vi "下载查询数据库.vi"(8 "时间标识":timestamp=timestamp(3675413438.482 s since 1904-01-01), 9 "Row name":string="13131", 10 "pathcheck选项":T1, 11 "数据库操作选项":T2) -> (0 "OK":bool, 1 "Columns":string[](array[string]), 2 "Results":string[][](array[string]), 3 "Tables":string[](array[string]))   [LabVIEW 2017]
uses:
  Sqlite/CBB/ReadAllData.vi
  <vilib>/Utility/file.llb/Write Delimited Spreadsheet (string).vi
  Sqlite/CBB/DeleteRow.vi
  Sqlite/SQLite.lvlib
  Sqlite/CBB/DropTable.vi
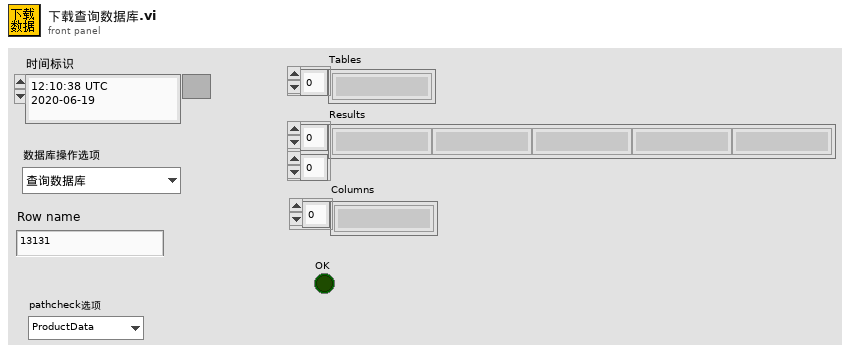
[diagram p1: front panel]
types:
  T1 = typedef "pathcheck选项.ctl" = enum16{"ProductData", "CTData", "ERData", "IOTDATA"}
  T2 = typedef "数据库操作选项.ctl" = enum16{"查询数据库", "下载数据", "删除table", "删除数据库对应行"}
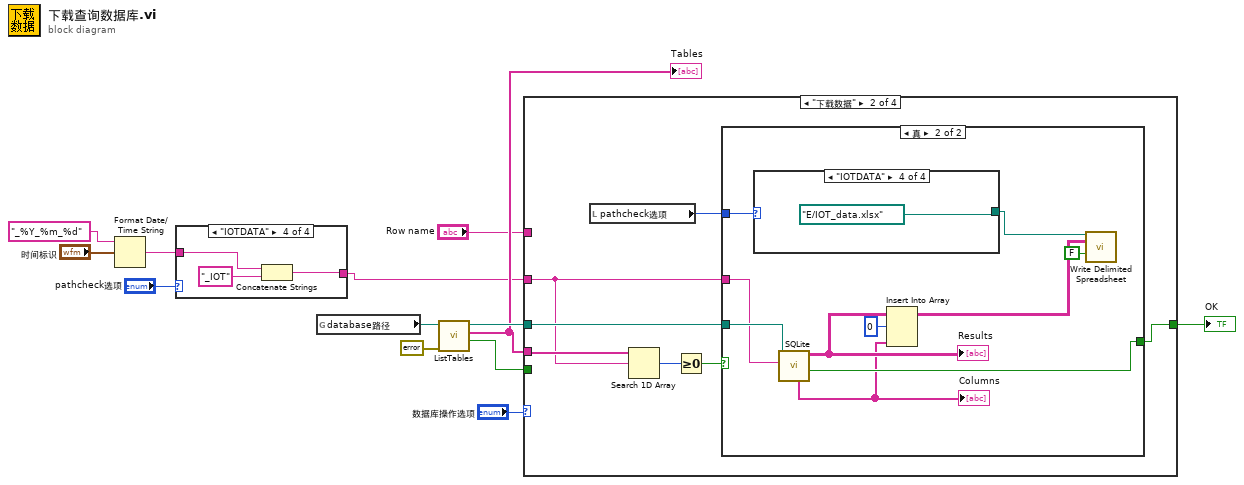
[diagram p0: block diagram]
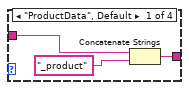
[diagram p2: hidden frame]
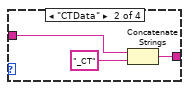
[diagram p3: hidden frame]
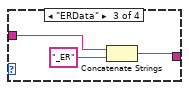
[diagram p4: hidden frame]
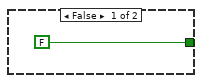
[diagram p6: hidden frame]
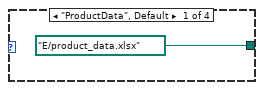
[diagram p7: hidden frame]
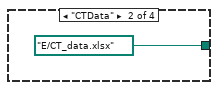
[diagram p8: hidden frame]
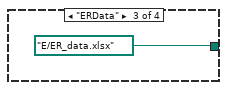
[diagram p9: hidden frame]
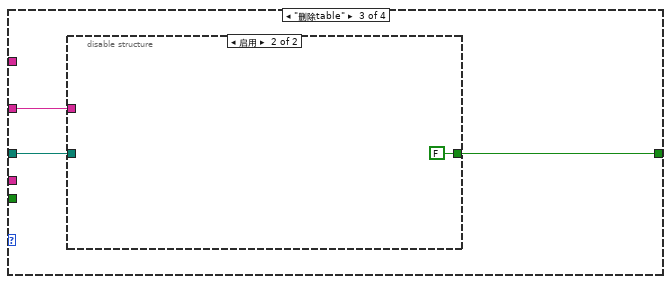
[diagram p10: hidden frame]
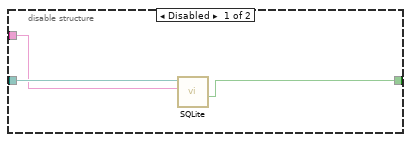
[diagram p11: hidden frame]
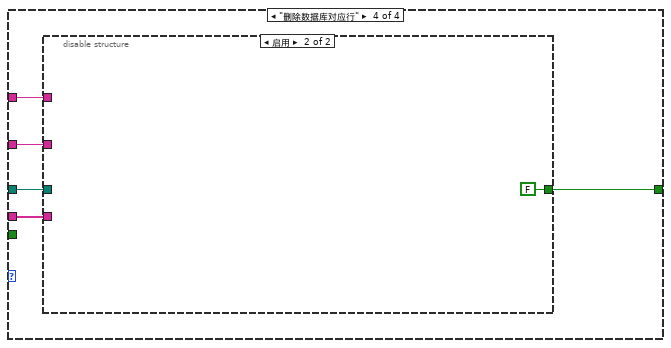
[diagram p12: hidden frame]
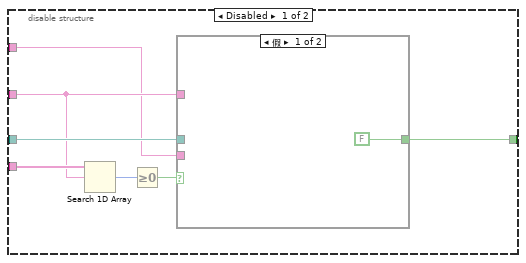
[diagram p13: hidden frame]
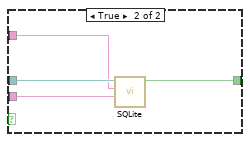
[diagram p14: hidden frame]
diagram:
  n1 = Format Date/Time String(time format string (%c)="_%Y_%m_%d" ("时间格式字符串(%c)"), seconds (now)="时间标识") -> (date/time string=w2:string)  [unwired: 1 in]
  n2 = case shown="\"IOTDATA\"" "pathcheck选项" {
    tunnel: w2 -> [w16 w18 w21 w24]
    tunnel: [w14 w17 w20 w23] -> w1
    frame "ProductData", Default {
      n3 = Concatenate Strings(w16, "_product" ("字符串")) -> (w14:string)
    }
    frame "CTData" {
      n4 = Concatenate Strings(w18, "_CT" ("字符串")) -> (w17:string)
    }
    frame "ERData" {
      n5 = Concatenate Strings(w21, "_ER" ("字符串")) -> (w20:string)
    }
    frame "IOTDATA" {
      n6 = Concatenate Strings(w24, "_IOT" ("字符串")) -> (w23:string)
    }
  }
  n7 = global read "数据库全局.vi" "database路径"() -> (w12:path)
  n8 = call "ListTables.vi"("error in (no error)"=errorcluster {"status"=FALSE, "code"=0, "source"=""}, "DbPath"=w12) -> ("OK？"=w4:bool, "Tables"=w7:string[], "DbPathout"=w10:path)  [unwired: 6 in, 1 out]
  "Tables" <- w7
  n9 = case shown="\"下载数据\"" "数据库操作选项" {
    tunnel: w10 -> [_ w33 w51 w59]
    tunnel: w7 -> [_ w31 _ w60]
    tunnel: w1 -> [_ w30 w50 w58]
    tunnel: "Row name" -> [_ _ _ w57]
    tunnel: [w26 w28 w49 w56] -> w5
    tunnel: w4 -> [w26 _ _ _]
    frame "查询数据库", Default {
    }
    frame "下载数据" {
      n10 = local read "pathcheck选项"() -> (w27:T1)
      n11 = Search 1D Array(1D array=w31, element=w30) -> (index of element=w32:i32)  [unwired: 1 in]
      n12 = Greater Or Equal To 0?(x=w32) -> (x >= 0?=w29:bool)
      n13 = case shown="真" w29 {
        tunnel: w33 -> [_ w44]
        tunnel: w30 -> [_ w43]
        tunnel: [FALSE ("OK") w42] -> w28
        tunnel: w27 -> [_ w36]
        frame False {
        }
        frame True {
          n14 = case shown="\"IOTDATA\"" w36 {
            tunnel: [path "E:/product_data.xlsx" path "E:/CT_data.xlsx" path "E:/ER_data.xlsx" path "E:/IOT_data.xlsx"] -> w35
            frame "ProductData", Default {
            }
            frame "CTData" {
            }
            frame "ERData" {
            }
            frame "IOTDATA" {
            }
          }
          n15 = call-poly "SQLite.vi"("Table Name"=w43, "DbPath"=w44) -> ("OK"=w42:bool, "Results"=w41:string[][], "Columns"=w39:string[])  [unwired: 4 in, 3 out]
          "Results" <- w41
          "Columns" <- w39
          n16 = Insert Into Array(array=w41, index (row)=0 ("索引 (行)"), new element=w39) -> (w38:string[][])  [unwired: 1 in]
          n17 = call-poly <vilib>:"Write Delimited Spreadsheet.vi"("file path (dialog if empty)"=w35, "2D data"=w38, "append to file? (new file:F)"=FALSE) -> ()  [unwired: 11 in, 2 out]
        }
      }
    }
    frame "删除table" {
      n18 = disable-structure shown="启用" {
        disable-tunnel: w51 -> [w54 _]
        disable-tunnel: w50 -> [w53 _]
        disable-tunnel: [w52 FALSE ("OK？")] -> w49
        frame Disabled {
          n19 = call-poly "SQLite.vi"("Table Name"=w53, "Path"=w54) -> ("OK？"=w52:bool)  [unwired: 7 in, 2 out]
        }
        frame Enabled {
        }
      }
    }
    frame "删除数据库对应行" {
      n20 = disable-structure shown="启用" {
        disable-tunnel: w60 -> [w66 _]
        disable-tunnel: w59 -> [w64 _]
        disable-tunnel: w58 -> [w63 _]
        disable-tunnel: w57 -> [w62 _]
        disable-tunnel: [w61 FALSE ("OK")] -> w56
        frame Disabled {
          n21 = Search 1D Array(1D array=w66, element=w63) -> (index of element=w67:i32)  [unwired: 1 in]
          n22 = Greater Or Equal To 0?(x=w67) -> (x >= 0?=w65:bool)
          n23 = case shown="假" w65 {
            tunnel: w64 -> [_ w72]
            tunnel: w63 -> [_ w71]
            tunnel: w62 -> [_ w70]
            tunnel: [FALSE ("OK") w69] -> w61
            frame False {
            }
            frame True {
              n24 = call-poly "SQLite.vi"("Frist ColData"=w70, "Table Name"=w71, "DbPath"=w72) -> ("OK"=w69:bool)  [unwired: 6 in, 2 out]
            }
          }
        }
        frame Enabled {
        }
      }
    }
  }
  "OK" <- w5
